vi "WriteConfiguration_Pane.vi"(7 "PythonConverter_GUI in":refnum<class "PythonConverter_GUI.lvclass">, 8 "error in":errorcluster, 11 "Pane in":refnum<class "Pane.lvclass">) -> (0 "error out":errorcluster, 3 "Pane out":refnum<class "Pane.lvclass">, 5 "PythonConverter_GUI out":refnum<class "PythonConverter_GUI.lvclass">)   [LabVIEW 2014, in "PythonConverter_GUI.lvclass"]
uses:
  PythonConverter_GUI.lvclass
  VI Interpreter/Classes/Pane/Pane.lvclass
  PythonConverter_GUI.lvclass/PythonConverter_GUI.ctl
  PythonConfiguration/PythonConfiguration.lvclass/PythonConfiguration.ctl
  VI Interpreter/Classes/Pane/Pane.lvclass/Pane.ctl
  VI Interpreter/Classes/GObject/GObject.lvclass/GObject.ctl
  PythonConfiguration/PythonConfiguration.lvclass
  VI Interpreter/Classes/GObject/GObject.lvclass
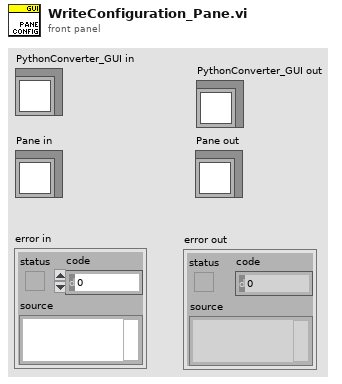
[diagram p1: front panel]
types:
  T1 = typedef "PythonConfiguration.lvclass/ItemTD.ctl" = cluster{"Key":string, "Value":string}
  T2 = typedef "LVBoundsTypeDef.ctl" = cluster{"Width":u32, "Height":u32}
  T3 = enum16{"Always On", "Always Off", "Off While Running"}
  T4 = typedef "LVPointTypeDef.ctl" = cluster{"Horizontal":i16, "Vertical":i16}
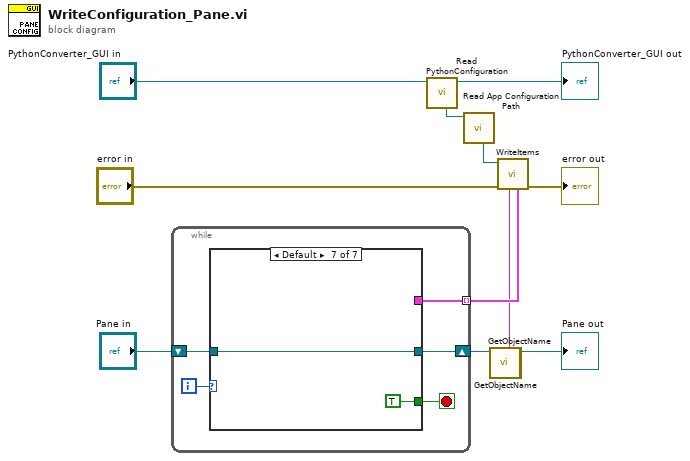
[diagram p0: block diagram]
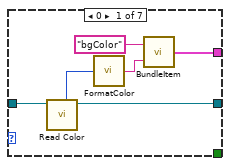
[diagram p2: hidden frame]
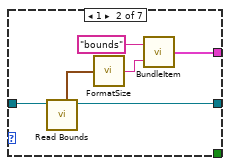
[diagram p3: hidden frame]
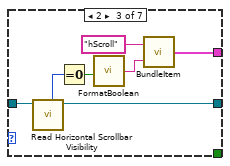
[diagram p4: hidden frame]
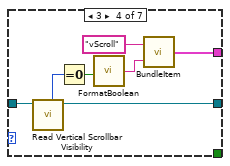
[diagram p5: hidden frame]
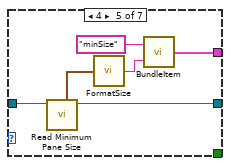
[diagram p6: hidden frame]
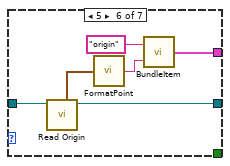
[diagram p7: hidden frame]
diagram:
  n1 = while {
    shift-right: [w14] -> w1
    shift-left: "Pane in" -> [w15]
    tunnel: [w13] -> w10 mode=indexing
    i -> [w16]
    stop <- w12 stop-if-true
    n2 = case shown="Default" w16 {
      tunnel: w15 -> [w19 w25 w33 w40 w45 w51 w56]
      tunnel: [w18 w24 w32 w39 w44 w50 w56] -> w14
      tunnel: [w17 w23 w31 w38 w43 w49 _] -> w13
      tunnel: [_ _ _ _ _ _ TRUE] -> w12
      frame 0 {
        n3 = call "Read Color.vi"("Pane in"=w19) -> ("Pane out"=w18:refnum<class "Pane.lvclass">, "Color"=w20:u32)  [unwired: 7 in]
        n4 = call "FormatColor.vi"("color"=w20) -> ("value"=w21:string)
        n5 = call "BundleItem.vi"("Value"=w21, "Key"="bgColor") -> ("Item"=w17:T1)
      }
      frame 1 {
        n6 = call "Read Bounds.vi"("GObject in"=w25) -> ("GObject out"=w24:refnum<class "Pane.lvclass">, "Bounds"=w26:T2)  [unwired: 7 in]
        n7 = call "FormatSize.vi"("size"=w26) -> ("value"=w27:string)
        n8 = call "BundleItem.vi"("Value"=w27, "Key"="bounds") -> ("Item"=w23:T1)
      }
      frame 2 {
        n9 = call "Read Horizontal Scrollbar Visibility.vi"("Pane in"=w33) -> ("Pane out"=w32:refnum<class "Pane.lvclass">, "Horizontal Scrollbar Visibility"=w29:T3)  [unwired: 7 in]
        n10 = Equal To 0?(x=w29) -> (x = 0?=w30:bool)
        n11 = call "FormatBoolean.vi"("boolean"=w30) -> ("value"=w34:string)
        n12 = call "BundleItem.vi"("Value"=w34, "Key"="hScroll") -> ("Item"=w31:T1)
      }
      frame 3 {
        n13 = call "Read Vertical Scrollbar Visibility.vi"("Pane in"=w40) -> ("Pane out"=w39:refnum<class "Pane.lvclass">, "Vertical Scrollbar Visibility"=w36:T3)  [unwired: 7 in]
        n14 = Equal To 0?(x=w36) -> (x = 0?=w37:bool)
        n15 = call "FormatBoolean.vi"("boolean"=w37) -> ("value"=w41:string)
        n16 = call "BundleItem.vi"("Value"=w41, "Key"="vScroll") -> ("Item"=w38:T1)
      }
      frame 4 {
        n17 = call "Read Minimum Pane Size.vi"("Pane in"=w45) -> ("Pane out"=w44:refnum<class "Pane.lvclass">, "Minimum Pane Size"=w46:T4)  [unwired: 7 in]
        n18 = call "FormatSize.vi"("size"=w46) -> ("value"=w47:string)
        n19 = call "BundleItem.vi"("Value"=w47, "Key"="minSize") -> ("Item"=w43:T1)
      }
      frame 5 {
        n20 = call "Read Origin.vi"("Pane in"=w51) -> ("Pane out"=w50:refnum<class "Pane.lvclass">, "Origin"=w52:T4)  [unwired: 7 in]
        n21 = call "FormatPoint.vi"("point"=w52) -> ("value"=w53:string)
        n22 = call "BundleItem.vi"("Value"=w53, "Key"="origin") -> ("Item"=w49:T1)
      }
      frame Default {
      }
    }
  }
  n23 = call "Read PythonConfiguration.vi"("PythonConverter_GUI in"="PythonConverter_GUI in") -> ("PythonConverter_GUI out"=→"PythonConverter_GUI out":refnum<class "PythonConverter_GUI.lvclass">, "PythonConfiguration"=w5:refnum<class "PythonConfiguration.lvclass">)  [unwired: 7 in]
  n24 = call "Read App Configuration Path.vi"("PythonConfiguration in"=w5) -> ("App Configuration Path"=w4:path)  [unwired: 7 in, 1 out]
  n25 = call-dynamic "GetObjectName.vi"("GObject in"=w1) -> ("GObject out"=→"Pane out":refnum<class "Pane.lvclass">, "Name"=w9:string)  [unwired: 6 in, 1 out]
  n26 = call-dynamic "GetObjectName.vi"("GObject in"=w1) -> ()  [unwired: 6 in, 3 out]
  n27 = call "WriteItems.vi"("Items"=w10, "section"=w9, "error in"="error in", "Path"=w4) -> ("error out"=→"error out":errorcluster)  [unwired: 5 in]
